vi "set parent queue for new connections.vi"(10 "conn parent queue":refnum<class "identifying queue.lvclass">, 11 "queue manager in":refnum<class "queue manager.lvclass">) -> (3 "queue manager out":refnum<class "queue manager.lvclass">)   [LabVIEW 2015, in "queue manager.lvclass"]
uses:
  queue manager.lvclass
  communicator queue/identifying queue.lvclass
  queue manager.lvclass/queue manager.ctl
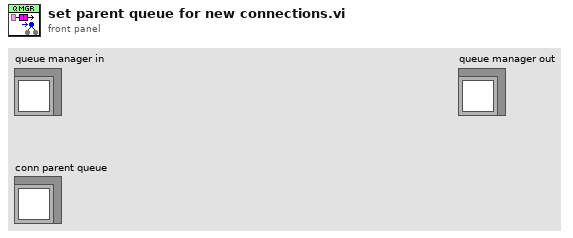
[diagram p1: front panel]
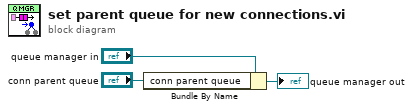
[diagram p0: block diagram]
diagram:
  n1 = Bundle By Name(cluster="queue manager in", "conn parent queue"="conn parent queue") -> (→"queue manager out":refnum<class "queue manager.lvclass">)
